vi "2_Analog_Meter_Reader(Training).vi"() -> ()   [LabVIEW 2020]
doc: "This example demonstrating the usage of Deep Learning toolkit for solving geometrical objects recognition problem based on Multilayer perceptron (MLP) and Convolutional Neural Network (CNN)."
uses:
  <vilib>/Ngene/DeepLTK/Toolkit/NN_Train/Controls/NN_LR_Policy_Cfg.ctl
  <vilib>/Ngene/DeepLTK/Toolkit/NN_Train/Controls/NN_LR_Policy_Type.ctl
  <vilib>/Ngene/DeepLTK/Toolkit/NN_Train/Controls/NN_Train_Params.ctl
  <vilib>/Ngene/DeepLTK/Toolkit/NN_Train/Controls/NN_Train_Optimizer.ctl
  <vilib>/Ngene/DeepLTK/Toolkit/NN_Train/Controls/NN_Train_Data_Sampling.ctl
  Controls/Regression_Report.ctl
  <vilib>/Ngene/DeepLTK/Toolkit/NN_Layers/Layers/FC/Controls/NN_Layer_Config(FC).ctl
  <vilib>/Ngene/DeepLTK/Toolkit/NN_Activations/Controls/NN_Activation_Type.ctl
  <vilib>/Ngene/DeepLTK/Toolkit/NN_Layers/Controls/NN_Layer_Init_Params.ctl
  <vilib>/Ngene/DeepLTK/Toolkit/NN_Layers/Controls/NN_Layer_Weight_Init_Type.ctl
  <vilib>/Ngene/DeepLTK/Toolkit/NN_Layers/Layers/Input/Controls/NN_Layer_Config(Input3D).ctl
  <vilib>/Ngene/DeepLTK/Toolkit/NN_Data/Controls/NN_Dims(C,H,W).ctl
  <vilib>/Ngene/DeepLTK/Toolkit/NN_Network/Controls/NN_Save_Before_Destroy_Options.ctl
  <vilib>/Ngene/DeepLTK/Toolkit/NN_Layers/Layers/Conv2D/Controls/NN_Layer_Config(Conv2D).ctl
  <vilib>/Ngene/DeepLTK/Toolkit/NN_Layers/Layers/Conv2D/Controls/NN_Layer_Params(Conv2D).ctl
  <vilib>/Ngene/DeepLTK/Toolkit/NN_Layers/Layers/Conv2D/Controls/NN_Conv2D_Padding_Type.ctl
  <vilib>/Ngene/DeepLTK/Toolkit/NN_Layers/Layers/DropOut3D/Controls/NN_Layer_Config(DropOut3D).ctl
  cd255efe-81e1-4e35-9bfd-5e2bf705b7ac.vi
  <vilib>/Ngene/DeepLTK/Toolkit/NN_Layers/Layers/Input/NN_Layer_Create(Input3D).vi
  <vilib>/Ngene/DeepLTK/Toolkit/NN_Layers/Layers/Conv2D/NN_Layer_Create(Conv2D).vi
  <vilib>/Ngene/DeepLTK/Toolkit/NN_Layers/Layers/DropOut3D/NN_Layer_Create(DropOut3D).vi
  <vilib>/Ngene/DeepLTK/Toolkit/NN_Layers/Layers/FC/NN_Layer_Create(FC).vi
  <vilib>/Ngene/DeepLTK/Toolkit/NN_Train/Loss_Functions/NN_Set_Loss(MSE).vi
  <vilib>/ptbypt/Filters.llb/FIR Filter PtByPt.vi
  <vilib>/Ngene/DeepLTK/Toolkit/NN_Network/subVIs/NN_Predict/NN_Predict(In3D_Out1D).vi
  <vilib>/Ngene/DeepLTK/Toolkit/NN_Train/Eval_Loss/NN_Eval_Test_Error_Loss/NN_Eval(In3D_Out1D).vi
  <vilib>/Ngene/DeepLTK/Toolkit/NN_Data/subVIs/Dataset_Destroy/NN_Datasets_All_Destroy(In3D_Out1D).vi
  <vilib>/Ngene/DeepLTK/Toolkit/Deep_Learning_Toolkit_by_Ngene.lvlib
panel:
  in  "BN Merge?":bool
  in  "NN Device":enum16{"CPU", "GPU"}(ring)=enum."GPU"
  out "Train Speed (img/s)":dbl=1309.0022539272923 format="%#_3p"
  out "Train Speed (sec/batch)":dbl=0.0488922000004095 format="%#_3p"
  out "Elapsed Time":dbl=45.66759789999924 format="%<%H:%M:%S>t"
  out "Test.Dataset_Size":i32=200
  out "Train.Dataset_Size":i32=1000
  out "Loss Values":cluster{"Train_Loss":dbl, "Test_Loss":dbl}={"Train_Loss"=31.746196746826172, "Test_Loss"=0.6291578412055969} {"Test_Loss" format="%#_4g"}
  out "Session Data":T1={"Epochs"=50.04800033569336, "Tot_Iter"=782.0, "LR"=1.5258789289873675e-06, "LR_iter"=783.0} {"LR" format="%#_3g"}
  out "Loss Charts":cluster{"Filtered x":sgl, "Test_Loss":sgl}(graph)={"Filtered x"=31.746197, "Test_Loss"=0.62915784}
  in  "Image Folder(Test)":path=path "D:/Data/DNN/_DeepLTK_Examples/Analog_Meter/Test/Images"
  in  "Labels (Test)":path=path "D:/Data/DNN/_DeepLTK_Examples/Analog_Meter/Test/Labels.csv"
  in  "Stop":bool
  out "Regression Metrics":T2={"Graphs"=[{"Best Linear Fit"=[0.0, 0.7035179734230042, 1.407034993171692, 2.110553026199341, 2.814069986343384, 3.517587900161743, 4.221106052398682, 4.924623012542725, 5.628140926361084, 6.331657886505127, 7.035175800323486, 7.7386932373046875, 8.442211151123047, 9.145729064941406, 9.84924602508545, 10.552763938903809, 11.256280899047852, 11.959798812866211, 12.66331672668457, 13.366833686828613, 14.070351600646973, 14.773868560791016, 15.477387428283691, 16.180904388427734, 16.884422302246094, 17.587940216064453, 18.29145622253418, 18.99497413635254, 19.6984920501709, 20.402009963989258, 21.105527877807617, 21.809045791625977, 22.512563705444336, 23.216079711914062, 23.919597625732422, 24.62311553955078, 25.32663345336914, 26.0301513671875, 26.733667373657227, 27.437185287475586, 28.140703201293945, 28.844221115112305, 29.547739028930664, 30.251256942749023, 30.954774856567383, 31.65829086303711, 32.36180877685547, 33.06532669067383, 33.76884460449219, 34.47236251831055, 35.175880432128906, 35.879398345947266, 36.582916259765625, 37.28643035888672, 37.98994827270508, 38.69346618652344, 39.3969841003418, 40.100502014160156, 40.804019927978516, 41.507537841796875, 42.211055755615234, 42.914573669433594, 43.61809158325195, 44.32160949707031, 45.02512741088867, 45.728641510009766, 46.432159423828125, 47.135677337646484, 47.839195251464844, 48.5427131652832, 49.24623107910156, 49.94974899291992, 50.65326690673828, 51.35678482055664, 52.060302734375, 52.76382064819336, 53.46733856201172, 54.17085266113281, 54.87437057495117, 55.57788848876953, 56.28140640258789, 56.98492431640625, 57.68844223022461, 58.39196014404297, 59.09547805786133, 59.79899597167969, 60.50251388549805, 61.206031799316406, 61.909549713134766, 62.61306381225586, 63.31658172607422, 64.02010345458984, 64.72361755371094, 65.42713928222656, 66.13065338134766, 66.83416748046875, 67.53768920898438, 68.24120330810547, 68.9447250366211, 69.64823913574219, 70.35176086425781, 71.0552749633789, 71.75879669189453, 72.46231079101562, 73.16583251953125, 73.86934661865234, 74.57286071777344, 75.27638244628906, 75.97989654541016, 76.68341827392578, 77.38693237304688, 78.0904541015625, 78.7939682006836, 79.49748992919922, 80.20100402832031, 80.90452575683594, 81.60803985595703, 82.31156158447266, 83.01507568359375, 83.71858978271484, 84.42211151123047, 85.12562561035156, 85.82914733886719, 86.53266143798828, 87.2361831665039, 87.939697265625, 88.64321899414062, 89.34673309326172, 90.05024719238281, 90.75376892089844, 91.45728302001953, 92.16080474853516, 92.86431884765625, 93.56784057617188, 94.27135467529297, 94.9748764038086, 95.67839050292969, 96.38191223144531, 97.0854263305664, 97.78894805908203, 98.49246215820312, 99.19597625732422, 99.89949798583984, 100.60301208496094, 101.30653381347656, 102.01004791259766, 102.71356964111328, 103.41708374023438, 104.12060546875, 104.8241195678711, 105.52764129638672, 106.23115539550781, 106.9346694946289, 107.63819122314453, 108.34170532226562, 109.04522705078125, 109.74874114990234, 110.45226287841797, 111.15577697753906, 111.85929870605469, 112.56281280517578, 113.2663345336914, 113.9698486328125, 114.67337036132812, 115.37688446044922, 116.08039855957031, 116.78392028808594, 117.48743438720703, 118.19095611572266, 118.89447021484375, 119.59799194335938, 120.30150604248047, 121.0050277709961, 121.70854187011719, 122.41206359863281, 123.1155776977539, 123.819091796875, 124.52261352539062, 125.22612762451172, 125.92964935302734, 126.63316345214844, 127.33668518066406, 128.0402069091797, 128.74371337890625, 129.44723510742188, 130.1507568359375, 130.85427856445312, 131.5577850341797, 132.2613067626953, 132.96482849121094, 133.6683349609375, 134.37185668945312, 135.07537841796875, 135.77890014648438, 136.48240661621094, 137.18592834472656, 137.8894500732422, 138.5929718017578, 139.29647827148438, 140.0], "Array 3"=[2.7411866, 2.7137148, 2.0073462, 1.9446042, 1.7734674, 5.416593, 5.3980837, 6.26864, 6.7600207, 8.353234, 8.55233, 9.980298, 10.729441, 9.132336, 10.401645, 11.213742, 11.992651, 12.844751, 14.88841, 15.243118, 15.098492, 15.378671, 15.892674, 16.883436, 17.707497, 18.54948, 19.383738, 19.991417, 20.575132, 21.72056, 22.378765, 22.813072, 23.103836, 23.772732, 24.9811, 26.010513, 26.093754, 26.587946, 27.25175, 28.095667, 28.975655, 29.689682, 30.23439, 31.040358, 31.723991, 32.394585, 33.01178, 33.938267, 34.69976, 35.091663, 36.21189, 36.8499, 37.374218, 37.59023, 37.901527, 40.05153, 40.292145, 40.65563, 41.26654, 41.888508, 42.676754, 43.337814, 44.55616, 44.666943, 45.762623, 46.638622, 47.10543, 47.582756, 48.254047, 48.7922, 48.93925, 50.20978, 51.65092, 52.034176, 52.772846, 53.44115, 53.83609, 54.339455, 54.967934, 56.191475, 56.93299, 57.32052, 57.90262, 58.44689, 59.871216, 60.415913, 61.335266, 61.844868, 62.402317, 63.24532, 63.46186, 63.923306, 64.566605, 65.41565, 66.25982, 67.834305, 68.40465, 69.21689, 69.92333, 69.99375, 70.9311, 71.24369, 71.90029, 72.55936, 73.256836, 74.641075, 75.15599, 76.08701, 76.65829, 77.369934, 77.71648, 78.54193, 79.1788, 79.38558, 80.159035, 80.798485, 82.40353, 83.0302, 83.6425, 84.09465, 84.48281, 85.91157, 86.571556, 87.207184, 87.52079, 88.28226, 88.86124, 89.166916, 90.6277, 91.75378, 92.084785, 92.846756, 93.38212, 94.035805, 94.30609, 95.19444, 96.14566, 96.334114, 97.50143, 97.97509, 98.78357, 99.17057, 99.90308, 100.55551, 100.895775, 103.138855, 103.663376, 103.84958, 104.11476, 104.78948, 105.572815, 106.37113, 107.03523, 108.05507, 108.38589, 108.887184, 109.62145, 110.51888, 111.377914, 112.20456, 113.260765, 113.89993, 114.512054, 114.628975, 114.61027, 115.974815, 117.448204, 118.181625, 118.56665, 118.8262, 119.137146, 120.336105, 121.32332, 121.78671, 122.472824, 123.28484, 123.92701, 124.72468, 125.16693, 125.67931, 126.1605, 126.6288, 128.87215, 129.15334, 129.38629, 130.32288, 131.47081, 129.8887, 131.07483, 132.84592, 133.95595, 134.20056, 135.08958, 136.01593, 136.3541, 139.61113, 139.59554, 138.77191, 139.19157, 138.16393]}, {"Best Linear Fit"=[1.703791476154765, 1.6760983977338209, 0.9640395930934129, 0.9007921830332941, 0.7282768621913387, 4.4007495436063815, 4.3820910541281295, 5.259660134609876, 5.754999120294974, 7.361046735724271, 7.561746268037751, 9.001217222822467, 9.756394553132358, 8.146424122116281, 9.425958025581274, 10.244597388811167, 11.029780581170945, 11.888745008143772, 13.948865858086812, 14.306431868754895, 14.160640218377182, 14.443076211129126, 14.961220497965941, 15.959963289813404, 16.79066191017369, 17.639428266384463, 18.480405711460797, 19.09298021121931, 19.681397742453232, 20.836052385556247, 21.499559557729306, 21.9373651966171, 22.23047128621935, 22.904755265824782, 24.12285752149887, 25.160563134793847, 25.244474183850688, 25.742647248778482, 26.41179950687865, 27.262513571551334, 28.149589988081473, 28.86936920719891, 29.418465330975305, 30.23092509401115, 30.92006587843905, 31.596061072783964, 32.21822798864954, 33.15217823004922, 33.91980608962376, 34.31486596886187, 35.44411772529289, 36.087265287492464, 36.615807607263136, 36.833558721505966, 37.14736474131641, 39.3146855038354, 39.5572396182348, 39.92365107093547, 40.53948456955176, 41.166462113819804, 41.96105794860334, 42.62744342242248, 43.855603390795714, 43.9672784183224, 45.07178485599256, 45.95484087924151, 46.425409550894265, 46.90658006307907, 47.58327897045169, 48.12576480627937, 48.27400214783531, 49.55476754909878, 51.00751579982002, 51.39385809745271, 52.13847877099053, 52.81216670950693, 53.2102875481442, 53.71770694080479, 54.35124862790496, 55.58464606700894, 56.332135428626884, 56.72278460380614, 57.309573596967766, 57.85823134213674, 59.29402895337113, 59.84311354086838, 60.769872834935846, 61.28357949972914, 61.845519347617625, 62.69531243267209, 62.91359806118186, 63.37876006334312, 64.02724123193296, 64.88312547237472, 65.73409525790173, 67.32126423319247, 67.89620162224826, 68.71498518896743, 69.42711970043972, 69.49810627143047, 70.44300444173648, 70.75811406109004, 71.42000423146995, 72.08437854729189, 72.78747630676914, 74.18286617759341, 74.70192952133524, 75.64045197470178, 76.21632764779451, 76.93370732085029, 77.28304123499353, 78.11514535869603, 78.7571469838341, 78.96559216623524, 79.74527543751378, 80.38987657088532, 82.0078474114868, 82.63956636648244, 83.25680344572774, 83.71259414379884, 84.10388165975732, 85.54414765644628, 86.2094525654524, 86.85020058159031, 87.16633308436117, 87.93393402595105, 88.51757746033311, 88.82571916708454, 90.29827136366724, 91.43341815874014, 91.76709349666051, 92.53520203453265, 93.07487686367593, 93.73382912830084, 94.00629296909061, 94.9018004829608, 95.86068062358763, 96.05065237765508, 97.22736823190512, 97.7048471347643, 98.51983911107193, 98.90995761741063, 99.64837177276974, 100.30605504668898, 100.64905938900932, 102.91020855522142, 103.43895468259026, 103.62665763509303, 103.89397629538519, 104.57413224107421, 105.36377516667919, 106.16852292710821, 106.8379732057529, 107.86602487611871, 108.19950794272003, 108.7048431142822, 109.4450261657765, 110.34968579443314, 111.21563736114, 112.04894125787331, 113.11365522335429, 113.75797179517365, 114.37502429395268, 114.49288661252618, 114.47402864155441, 115.84956842140066, 117.33482590674573, 118.07415527358349, 118.4622818490569, 118.72392466001091, 119.03737305516793, 120.24599056667361, 121.24115615063027, 121.70828316567217, 122.39992155453444, 123.21848208652352, 123.86582116347824, 124.66991520142251, 125.11573086346165, 125.6322408440866, 126.11730292776883, 126.58937516113652, 128.85079350719525, 129.13424757658154, 129.36908007480815, 130.31320915983798, 131.47039024807324, 129.87553811087352, 131.071219608034, 132.85657416814172, 133.9755470998567, 134.22213122110324, 135.11831553001645, 136.05212349064004, 136.39301284845092, 139.67628403754952, 139.66056393450455, 138.83030561546488, 139.25334866247653, 138.2174215588827], "Array 3"=[2.7411866, 2.7137148, 2.0073462, 1.9446042, 1.7734674, 5.416593, 5.3980837, 6.26864, 6.7600207, 8.353234, 8.55233, 9.980298, 10.729441, 9.132336, 10.401645, 11.213742, 11.992651, 12.844751, 14.88841, 15.243118, 15.098492, 15.378671, 15.892674, 16.883436, 17.707497, 18.54948, 19.383738, 19.991417, 20.575132, 21.72056, 22.378765, 22.813072, 23.103836, 23.772732, 24.9811, 26.010513, 26.093754, 26.587946, 27.25175, 28.095667, 28.975655, 29.689682, 30.23439, 31.040358, 31.723991, 32.394585, 33.01178, 33.938267, 34.69976, 35.091663, 36.21189, 36.8499, 37.374218, 37.59023, 37.901527, 40.05153, 40.292145, 40.65563, 41.26654, 41.888508, 42.676754, 43.337814, 44.55616, 44.666943, 45.762623, 46.638622, 47.10543, 47.582756, 48.254047, 48.7922, 48.93925, 50.20978, 51.65092, 52.034176, 52.772846, 53.44115, 53.83609, 54.339455, 54.967934, 56.191475, 56.93299, 57.32052, 57.90262, 58.44689, 59.871216, 60.415913, 61.335266, 61.844868, 62.402317, 63.24532, 63.46186, 63.923306, 64.566605, 65.41565, 66.25982, 67.834305, 68.40465, 69.21689, 69.92333, 69.99375, 70.9311, 71.24369, 71.90029, 72.55936, 73.256836, 74.641075, 75.15599, 76.08701, 76.65829, 77.369934, 77.71648, 78.54193, 79.1788, 79.38558, 80.159035, 80.798485, 82.40353, 83.0302, 83.6425, 84.09465, 84.48281, 85.91157, 86.571556, 87.207184, 87.52079, 88.28226, 88.86124, 89.166916, 90.6277, 91.75378, 92.084785, 92.846756, 93.38212, 94.035805, 94.30609, 95.19444, 96.14566, 96.334114, 97.50143, 97.97509, 98.78357, 99.17057, 99.90308, 100.55551, 100.895775, 103.138855, 103.663376, 103.84958, 104.11476, 104.78948, 105.572815, 106.37113, 107.03523, 108.05507, 108.38589, 108.887184, 109.62145, 110.51888, 111.377914, 112.20456, 113.260765, 113.89993, 114.512054, 114.628975, 114.61027, 115.974815, 117.448204, 118.181625, 118.56665, 118.8262, 119.137146, 120.336105, 121.32332, 121.78671, 122.472824, 123.28484, 123.92701, 124.72468, 125.16693, 125.67931, 126.1605, 126.6288, 128.87215, 129.15334, 129.38629, 130.32288, 131.47081, 129.8887, 131.07483, 132.84592, 133.95595, 134.20056, 135.08958, 136.01593, 136.3541, 139.61113, 139.59554, 138.77191, 139.19157, 138.16393]}, {"Best Linear Fit"=[0.0, 140.0], "Array 3"=[0.0, 140.0]}], "y=k*x+b"="y = 0.992*x + 1.051", "R"=0.9999145, "R^2"=0.99982905, "MAE"=0.60552907, "MSE"=0.6291579} {"R" format="%#_7g"}
  in  "Evaluate Model":bool=TRUE
  in  "LR Update Policy":T3={"Policy_Type"=enum."Step", "LR0"=0.09999999999999964, "k"=3.0, "WarmUp_Policy"=enum."Ramp", "WarmUp_Iter"=50, "WarmUp_Ratio"=50.0} {"WarmUp_Ratio" min=1; "WarmUp_Iter" min=1; "LR0" format="%.7f"}
  in  "Train_Params":T5={"Optimizer"=enum."SGD", "Beta_1"=0.9, "Beta_2"=0.999, "Weight Decay(L1)"=0.0, "Weight Decay(L2)"=5e-08, "Data_Sampling"=enum."Random"}
  in  "Image Folder(Train)":path=path "D:/Data/DNN/_DeepLTK_Examples/Analog_Meter/Train/Images"
  in  "Labels (Train)":path=path "D:/Data/DNN/_DeepLTK_Examples/Analog_Meter/Train/Labels.csv"
  in  "Max_Epochs_to_Train":sgl=50.0
  in  "Input Height":i32=256
  in  "Input Width":i32=256
  out "Test_Loss":sgl=0.62915784
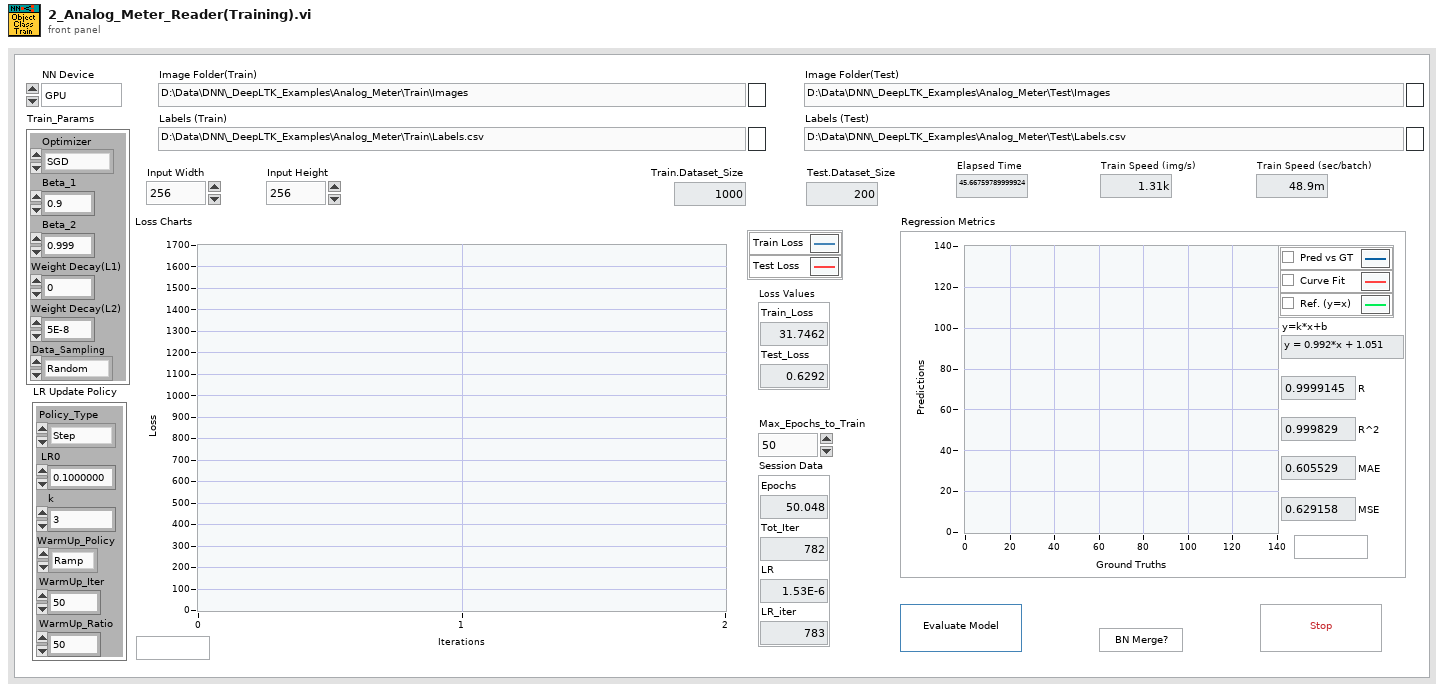
[diagram p1: front panel]
types:
  T1 = cluster{"Epochs":dbl, "Tot_Iter":dbl, "LR":dbl, "LR_iter":dbl}
  T2 = typedef "Regression_Report.ctl" = cluster{"Graphs":cluster{"Best Linear Fit":dbl[], "Array 3":sgl[]}[], "y=k*x+b":string, "R":sgl, "R^2":sgl, "MAE":sgl, "MSE":sgl}
  T3 = typedef "Deep_Learning_Toolkit_by_Ngene.lvlib/NN_LR_Policy_Cfg.ctl" = cluster{"Policy_Type":T4, "LR0":dbl, "k":sgl, "WarmUp_Policy":enum16{"Step", "Ramp"}, "WarmUp_Iter":i32, "WarmUp_Ratio":sgl}
  T4 = typedef "Deep_Learning_Toolkit_by_Ngene.lvlib/NN_LR_Policy_Type.ctl" = enum16{"Manual", "Step", "Exp", "1/t"}
  T5 = typedef "Deep_Learning_Toolkit_by_Ngene.lvlib/NN_Train_Params.ctl" = cluster{"Optimizer":T6, "Beta_1":sgl, "Beta_2":sgl, "Weight Decay(L1)":sgl, "Weight Decay(L2)":sgl, "Data_Sampling":T7}
  T6 = typedef "Deep_Learning_Toolkit_by_Ngene.lvlib/NN_Train_Optimizer.ctl" = enum16{"SGD", "Adam", "Adagrad", "Adadelta", "RMSProp", "Nesterov"}
  T7 = typedef "Deep_Learning_Toolkit_by_Ngene.lvlib/NN_Train_Data_Sampling.ctl" = enum16{"Random", "Sequential"}
  T8 = typedef "Deep_Learning_Toolkit_by_Ngene.lvlib/NN_Layer_Config(DropOut3D).ctl" = cluster{"Name":string, "Probability":sgl}
  T9 = typedef "Deep_Learning_Toolkit_by_Ngene.lvlib/NN_Layer_Config(FC).ctl" = cluster{"Name":string, "Size":i32, "BN":bool, "Activation":T10, "Init_Params":T11, "Custom_Params":string}
  T10 = typedef "Deep_Learning_Toolkit_by_Ngene.lvlib/NN_Activation_Type.ctl" = enum16{"Sigmoid", "ReLU", "LReLU", "ReLU6", "tanh", "Swish", "Mish", "None"}
  T11 = typedef "Deep_Learning_Toolkit_by_Ngene.lvlib/NN_Layer_Init_Params.ctl" = cluster{"Init_Type":T12, "Value":sgl}
  T12 = typedef "Deep_Learning_Toolkit_by_Ngene.lvlib/NN_Layer_Weight_Init_Type.ctl" = enum16{"Const", "Uniform", "Gaussian", "Xavier"}
  T13 = typedef "Deep_Learning_Toolkit_by_Ngene.lvlib/NN_Layer_Config(Conv2D).ctl" = cluster{"Name":string, "Conv_Params":T14, "BN?":bool, "Activation":T10, "Init_Params":T11, "Custom_Params":string}
  T14 = typedef "Deep_Learning_Toolkit_by_Ngene.lvlib/NN_Layer_Params(Conv2D).ctl" = cluster{"Filters":i32, "Kernel_Size":i32, "Stride":i32, "Pad_Type":T15, "Pad_Size":i32}
  T15 = typedef "Deep_Learning_Toolkit_by_Ngene.lvlib/NN_Conv2D_Padding_Type.ctl" = enum16{"Pad_Size", "Valid", "Same"}
  T16 = typedef "Deep_Learning_Toolkit_by_Ngene.lvlib/NN_Save_Before_Destroy_Options.ctl" = cluster{"CFG?":bool, "Weights?":bool, "Render?":bool}
  T17 = typedef "Deep_Learning_Toolkit_by_Ngene.lvlib/NN_Layer_Config(Input3D).ctl" = cluster{"Name":string, "Dims":T18}
  T18 = typedef "Deep_Learning_Toolkit_by_Ngene.lvlib/NN_Dims(C,H,W).ctl" = cluster{"C":i32, "H":i32, "W":i32}
  T19 = typedef "Deep_Learning_Toolkit_by_Ngene.lvlib/NN_DataSets_All(In3D_Out1D).ctl" = cluster{"Train":T20, "Validation":T20, "Test":T20}
  T20 = typedef "Deep_Learning_Toolkit_by_Ngene.lvlib/NN_DataSet(In3D_Out1D).ctl" = cluster{"Inputs Ref.":T21, "Outputs Ref.":T22, "Dataset_Size":i32, "Outputs_idx Ref.":T23, "Dims_In":T18, "Dims_Out":i32, "Labels":string[], "File Paths":path[]}
  T21 = typedef "Deep_Learning_Toolkit_by_Ngene.lvlib/NN_Data_ref(4D_SGL).ctl" = refnum<data-value>
  T22 = typedef "Deep_Learning_Toolkit_by_Ngene.lvlib/NN_Data_ref(2D_SGL).ctl" = refnum<data-value>
  T23 = typedef "Deep_Learning_Toolkit_by_Ngene.lvlib/NN_Data_ref(1D_I32).ctl" = refnum<data-value>
  T24 = typedef "Deep_Learning_Toolkit_by_Ngene.lvlib/NN.ctl" = cluster{"Name":string, "No of Layers":i32, "mBatch":i32, "Layers":T25[], "Dimty":T26, "Dims_In":T18, "Dims_Out":T18, "Working_Dir":path, "Train?":bool, "Train_Params":T5, "LR_Update_Policy":T3, "Session Data":T27, "Ground_truth":T28, "NNg_hdls":T29, "NN_Device":T30, "GPU Id":i32, "Labels":string[], "Receptive Field":T31[], "Loss_Type":T32, "Loss_Cfg_Prms":variant}
  T25 = typedef "Deep_Learning_Toolkit_by_Ngene.lvlib/NN_Layer_ref.ctl" = refnum<data-value>
  T26 = typedef "Deep_Learning_Toolkit_by_Ngene.lvlib/NN_In_Out_Dim-ty.ctl" = enum8{"In1D_Out1D", "In3D_Out1D", "In3D_Out3D", "In3D_OutBBox"}
  T27 = typedef "Deep_Learning_Toolkit_by_Ngene.lvlib/NN_Train_Session_Data.ctl" = cluster{"Epochs":sgl, "Tot_Iter":i32, "LR":sgl, "LR_iter":i32}
  T28 = typedef "Deep_Learning_Toolkit_by_Ngene.lvlib/NN_Ground_truth.ctl" = cluster{"Y":variant, "Y_idx":T23}
  T29 = typedef "Deep_Learning_Toolkit_by_Ngene.lvlib/nng_cuda_handles.ctl" = cluster{"cudnn":u64, "cublas":u64, "stream":u64, "curand":u64}
  T30 = typedef "Deep_Learning_Toolkit_by_Ngene.lvlib/NN_Device.ctl" = enum16{"CPU", "GPU"}
  T31 = typedef "Deep_Learning_Toolkit_by_Ngene.lvlib/NN_Dims(V,H).ctl" = cluster{"V":i32, "H":i32}
  T32 = typedef "Deep_Learning_Toolkit_by_Ngene.lvlib/NN_Loss_Type.ctl" = enum16{"None", "MSE", "CrossEntropy", "YOLO_v2"}
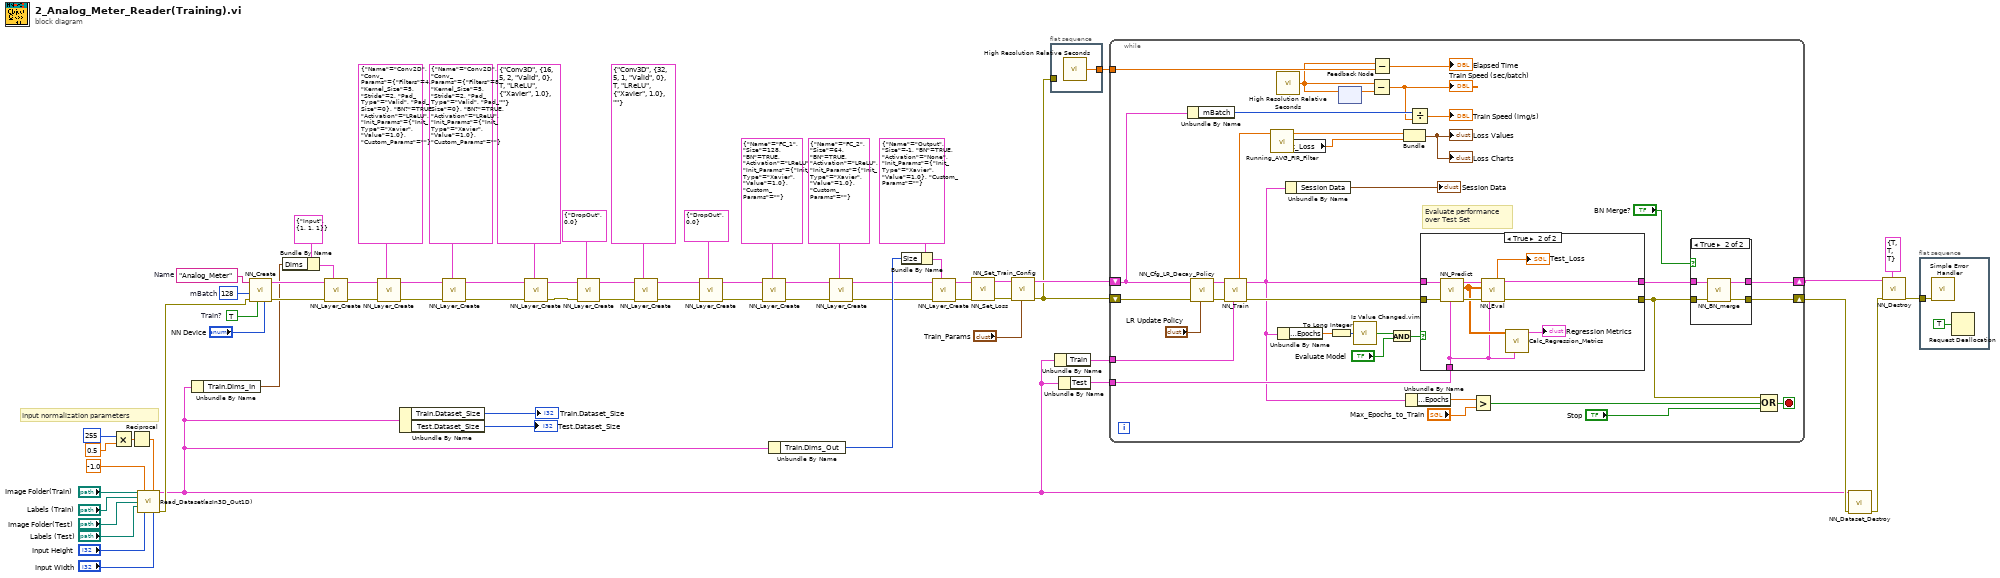
[diagram p0: block diagram]
diagram:
  w50 = TRUE  # Train?
  w62 = 128  # mBatch
  w67 = "Analog_Meter"  # Name
  # "Input normalization parameters"
  n1 = Multiply(x=u16 255 ("Shift"), y=sgl 0.5 ("Scale")) -> (x*y=w23:sgl)
  n2 = Reciprocal(x=w23) -> (1/x=w22:sgl)
  n3 = call "Read_Dataset(asIn3D_Out1D).vi"("Image Folder Path(Train)"="Image Folder(Train)", "Norm. Shift"=sgl -1.0 ("Scale"), "Norm. Scale"=w22, "Label File Path(Train)"="Labels (Train)", "Image Folder Path(Test)"="Image Folder(Test)", "Label File Path(Test)"="Labels (Test)", "Img Heigth"="Input Height", "Img Width"="Input Width") -> ("Datasets"=w17:T19, "error out"=w68:errorcluster)  [unwired: 6 in]
  n4 = Unbundle By Name(w17) -> ("Train.Dims_In"=w45:T18)
  n5 = call <vilib>:"NN_Create.vi"("NN_Device"="NN Device", "Train? (false)"=w50, "error in (no error)"=w68, "mBatch (1)"=w62, "Name"=w67) -> ("error out"=w65:errorcluster, "NN out"=w66:T24)  [unwired: 5 in]
  n6 = Bundle By Name(cluster=T17 {"Name"="Input", "Dims"={"C"=1, "H"=1, "W"=1}} ("Cluster"), "Dims"=w45) -> (w53:T17)
  n7 = call-poly <vilib>:"NN_Layer_Create.vi"("Input3D_Cfg"=w53, "error in (no error)"=w65, "NN In"=w66) -> ("error out"=w59:errorcluster, "NN out"=w60:T24)  [unwired: 6 in, 1 out]
  n8 = call-poly <vilib>:"NN_Layer_Create.vi"("Conv2D_Cfg"=T13 {"Name"="Conv2D", "Conv_Params"={"Filters"=4, "Kernel_Size"=5, "Stride"=2, "Pad_Type"=enum."Valid", "Pad_Size"=0}, "BN?"=TRUE, "Activation"=enum."LReLU", "Init_Params"={"Init_Type"=enum."Xavier", "Value"=1.0}, "Custom_Params"=""}, "error in (no error)"=w59, "NN in"=w60) -> ("error out"=w19:errorcluster, "NN out"=w18:T24)  [unwired: 6 in, 1 out]
  n9 = Unbundle By Name(w17) -> ("Train.Dataset_Size"=→"Train.Dataset_Size":i32, "Test.Dataset_Size"=→"Test.Dataset_Size":i32)
  n10 = call-poly <vilib>:"NN_Layer_Create.vi"("Conv2D_Cfg"=T13 {"Name"="Conv2D", "Conv_Params"={"Filters"=8, "Kernel_Size"=5, "Stride"=2, "Pad_Type"=enum."Valid", "Pad_Size"=0}, "BN?"=TRUE, "Activation"=enum."LReLU", "Init_Params"={"Init_Type"=enum."Xavier", "Value"=1.0}, "Custom_Params"=""}, "error in (no error)"=w19, "NN in"=w18) -> ("error out"=w42:errorcluster, "NN out"=w43:T24)  [unwired: 6 in, 1 out]
  n11 = call-poly <vilib>:"NN_Layer_Create.vi"("Conv2D_Cfg"=T13 {"Name"="Conv3D", "Conv_Params"={"Filters"=16, "Kernel_Size"=5, "Stride"=2, "Pad_Type"=enum."Valid", "Pad_Size"=0}, "BN?"=TRUE, "Activation"=enum."LReLU", "Init_Params"={"Init_Type"=enum."Xavier", "Value"=1.0}, "Custom_Params"=""}, "error in (no error)"=w42, "NN in"=w43) -> ("error out"=w8:errorcluster, "NN out"=w9:T24)  [unwired: 6 in, 1 out]
  n12 = call-poly <vilib>:"NN_Layer_Create.vi"("DropOut3D_Cfg"=T8 {"Name"="DropOut", "Probability"=0.0}, "error in (no error)"=w8, "NN in"=w9) -> ("error out"=w6:errorcluster, "NN out"=w7:T24)  [unwired: 6 in, 1 out]
  n13 = call-poly <vilib>:"NN_Layer_Create.vi"("Conv2D_Cfg"=T13 {"Name"="Conv3D", "Conv_Params"={"Filters"=32, "Kernel_Size"=5, "Stride"=1, "Pad_Type"=enum."Valid", "Pad_Size"=0}, "BN?"=TRUE, "Activation"=enum."LReLU", "Init_Params"={"Init_Type"=enum."Xavier", "Value"=1.0}, "Custom_Params"=""}, "error in (no error)"=w6, "NN in"=w7) -> ("error out"=w4:errorcluster, "NN out"=w5:T24)  [unwired: 6 in, 1 out]
  n14 = call-poly <vilib>:"NN_Layer_Create.vi"("DropOut3D_Cfg"=T8 {"Name"="DropOut", "Probability"=0.0}, "error in (no error)"=w4, "NN in"=w5) -> ("error out"=w2:errorcluster, "NN out"=w3:T24)  [unwired: 6 in, 1 out]
  n15 = call-poly <vilib>:"NN_Layer_Create.vi"("FC_Cfg"=T9 {"Name"="FC_1", "Size"=128, "BN"=TRUE, "Activation"=enum."LReLU", "Init_Params"={"Init_Type"=enum."Xavier", "Value"=1.0}, "Custom_Params"=""} ("Layer_Config_Params"), "error in (no error)"=w2, "NN in"=w3) -> ("error out"=w20:errorcluster, "NN out"=w21:T24)  [unwired: 6 in, 1 out]
  n16 = Unbundle By Name(w17) -> ("Train.Dims_Out"=w44:i32)
  n17 = call-poly <vilib>:"NN_Layer_Create.vi"("FC_Cfg"=T9 {"Name"="FC_2", "Size"=64, "BN"=TRUE, "Activation"=enum."LReLU", "Init_Params"={"Init_Type"=enum."Xavier", "Value"=1.0}, "Custom_Params"=""} ("Layer_Config_Params"), "error in (no error)"=w20, "NN in"=w21) -> ("error out"=w25:errorcluster, "NN out"=w26:T24)  [unwired: 6 in, 1 out]
  n18 = Bundle By Name(cluster=T9 {"Name"="Output", "Size"=-1, "BN"=TRUE, "Activation"=enum."None", "Init_Params"={"Init_Type"=enum."Xavier", "Value"=1.0}, "Custom_Params"=""} ("Layer_Config_Params"), "Size"=w44) -> (w54:T9)
  n19 = call-poly <vilib>:"NN_Layer_Create.vi"("FC_Cfg"=w54, "error in (no error)"=w25, "NN in"=w26) -> ("error out"=w57:errorcluster, "NN out"=w58:T24)  [unwired: 6 in, 1 out]
  n20 = call-poly <vilib>:"NN_Set_Loss.vi"("error in (no error)"=w57, "NN in"=w58) -> ("error out"=w37:errorcluster, "NN out"=w38:T24)  [unwired: 8 in]
  n21 = call <vilib>:"NN_Set_Train_Config.vi"("NN_Train_Params"="Train_Params", "error in (no error)"=w37, "NN in"=w38) -> ("error out"=w51:errorcluster, "NN out"=w52:T24)  [unwired: 7 in]
  n22 = flat-sequence {
    tunnel: [w69] -> w64
    tunnel: w51 -> [_]
    frame #0 {
      n23 = call <vilib>:"High Resolution Relative Seconds.vi"() -> ("relative seconds"=w69:dbl)
    }
  }
  n24 = Unbundle By Name(w17) -> ("Train"=w48:T20)
  n25 = Unbundle By Name(w17) -> ("Test"=w61:T20)
  n26 = while {
    shift-right: [w70] -> w36
    shift-left: w51 -> [w90]
    shift-right: [w73] -> w35
    shift-left: w52 -> [w91]
    tunnel: w64 -> [w97]
    tunnel: w48 -> [w82]
    tunnel: w61 -> [w93]
    stop <- w103 stop-if-true
    # "Evaluate performance \nover Test Set"
    n27 = Unbundle By Name(w91) -> ("mBatch"=w95:i32)
    n28 = call <vilib>:"NN_Cfg_LR_Decay_Policy.vi"("LR_Decay_Params"="LR Update Policy", "error in (no error)"=w90, "NN in"=w91) -> ("error out"=w98:errorcluster, "NN out"=w104:T24)  [unwired: 7 in]
    n29 = call <vilib>:"NN_Train.vi"("Train Dataset"=w82, "error in (no error)"=w98, "NN in"=w104) -> ("error out"=w94:errorcluster, "NN out"=w87:T24, "Loss"=w99:sgl)  [unwired: 5 in, 1 out]
    n30 = call <vilib>:"Running_AVG_FIR_Filter.vi"("Numeric"=w99) -> ("Filtered x"=w100:sgl)  [unwired: 10 in]
    n31 = local read "Test_Loss"() -> (w102:sgl)
    n32 = call <vilib>:"High Resolution Relative Seconds.vi"() -> ("relative seconds"=w96:dbl)
    n33 = Unbundle By Name(w87) -> ("Session Data.Epochs"=w86:sgl)
    n34 = Unbundle By Name(w87) -> ("Session Data"=→"Session Data":T27)
    n35 = To Long Integer(number=w86) -> (32bit integer=w85:i32)
    n36 = feedback #1() -> (w105:dbl)  [unwired: 1 in]
    n37 = feedback-in #1(w96) -> ()
    n38 = call "Is Value Changed.vim"("value"=w85) -> ("changed or first call?"=w83:bool)
    n39 = Subtract(x=w96, y=w105) -> (x-y=w76:dbl)
    "Train Speed (sec/batch)" <- w76
    n40 = Subtract(x=w96, y=w97) -> (x-y=→"Elapsed Time":dbl)
    n41 = And(x=w83, y="Evaluate Model") -> (x .and. y?=w84:bool)
    n42 = Bundle("Filtered x"=w100, "Test_Loss"=w102) -> (→"Loss Values" →"Loss Charts":cluster{"Filtered x":sgl, "Test_Loss":sgl})  [unwired: 1 in]
    n43 = Unbundle By Name(w87) -> ("Session Data.Epochs"=w88:sgl)
    n44 = Divide(x=w95, y=w76) -> (x/y=→"Train Speed (img/s)":dbl)
    n45 = case shown="True" w84 {
      tunnel: w87 -> [w112 w123]
      tunnel: w94 -> [w113 w118]
      tunnel: [w113 w120] -> w71
      tunnel: w93 -> [_ w114]
      tunnel: [w112 w121] -> w81
      frame False {
      }
      frame True {
        n46 = call-poly <vilib>:"NN_Predict.vi"("Dataset"=w114, "error in (no error)"=w118, "NN in"=w123) -> ("error out"=w117:errorcluster, "Predictions"=w116:sgl[][], "NN out"=w119:T24)  [unwired: 6 in]
        n47 = call-poly <vilib>:"NN_Eval.vi"("NN in"=w119, "Predictions"=w116, "error in (no error)"=w117, "Dataset"=w114) -> ("Loss"=→"Test_Loss":sgl, "NN out"=w121:T24, "error out"=w120:errorcluster)  [unwired: 7 in, 2 out]
        n48 = call "Calc_Regression_Metrics.vi"("Dataset"=w114, "Predictions"=w116) -> ("Metrics"=→"Regression Metrics":T2)  [unwired: 9 in]
      }
    }
    n49 = Greater?(x=w88, y="Max_Epochs_to_Train") -> (0:w79:bool)
    n50 = case shown="True" "BN Merge?" {
      tunnel: w81 -> [w107 w111]
      tunnel: [w107 w110] -> w73
      tunnel: w71 -> [w106 w109]
      tunnel: [w106 w108] -> w70
      frame False {
      }
      frame True {
        n51 = call <vilib>:"NN_BN_merge.vi"("error in (no error)"=w109, "NN in"=w111) -> ("error out"=w108:errorcluster, "NN out"=w110:T24)  [unwired: 8 in]
      }
    }
    n52 = Compound Arithmetic op=OR(w71, w79, "Stop") -> (w103:bool)
  }
  n53 = call-poly <vilib>:"NN_Dataset_Destroy.vi"("error in (no error)"=w36, "Datasets_All(In3D_Out1D)"=w17) -> ("error out"=w34:errorcluster)  [unwired: 9 in]
  n54 = call <vilib>:"NN_Destroy.vi"("Save (T, T, T)"=T16 {"CFG?"=TRUE, "Weights?"=TRUE, "Render?"=TRUE} ("Save_Config"), "error in (no error)"=w34, "NN in"=w35) -> ("error out"=w46:errorcluster)  [unwired: 8 in]
  n55 = flat-sequence {
    tunnel: w46 -> [w125]
    frame #0 {
      n56 = call <vilib>:"Simple Error Handler.vi"("error in (no error)"=w125) -> ()  [unwired: 4 in, 5 out]
      n57 = Request Deallocation(TRUE ("flag")) -> ()
    }
  }
